vi "Test Clip.vi"() -> ()   [LabVIEW 2019, in "DAQmx.lvclass"]
uses:
  DAQmx.lvclass
  typedefs/DAQ.Config.AO.Range--enum.ctl
  <vilib>/measure/NI_MABase.lvlib
  <resource>/objmgr/daqmx.rc
panel:
  in  "AO.Range":T1
  in  "amplitude":dbl=1.0 format="%0.2p"
  in  "Numeric":i32=1
  out "x-y":dbl
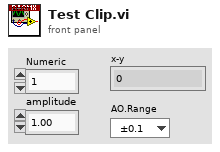
[diagram p1: front panel]
types:
  T1 = typedef "DAQmx.lvclass/DAQ.Config.AO.Range--enum.ctl" = enum16{"±0.1", "±1.0", "±3.5", "±10.0", ""}
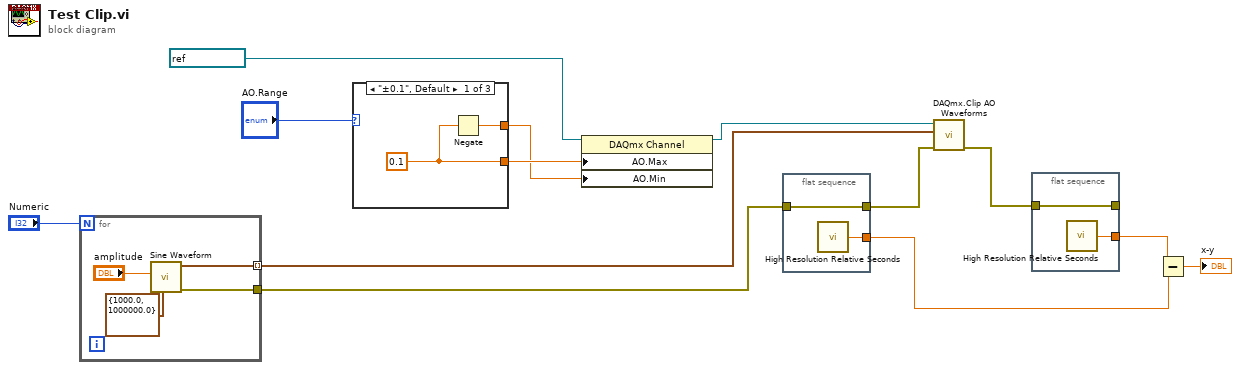
[diagram p0: block diagram]
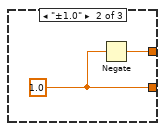
[diagram p2: hidden frame]
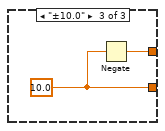
[diagram p3: hidden frame]
diagram:
  n1 = for {
    N: "Numeric" -> [_]
    tunnel: [w16] -> w11
    tunnel: [w15] -> w10 mode=indexing
    n2 = call <vilib>:"Sine Waveform.vi"("sampling info"=cluster{"Fs":dbl, "#s":dbl} {"Fs"=1000.0, "#s"=1000000.0}, "amplitude"="amplitude") -> ("error out"=w16:errorcluster, "signal out"=w15:waveform(dbl))  [unwired: 8 in]
  }
  n3 = case shown="\"±0.1\", Default" "AO.Range" {
    tunnel: [w19 w21 w23] -> w3
    tunnel: [w18 w20 w22] -> w2
    frame "±0.1", Default {
      w19 = 0.1
      n4 = Negate(x=w19) -> (-x=w18:dbl)
    }
    frame "±1.0" {
      w21 = 1.0
      n5 = Negate(x=w21) -> (-x=w20:dbl)
    }
    frame "±10.0" {
      w23 = 10.0
      n6 = Negate(x=w23) -> (-x=w22:dbl)
    }
  }
  n7 = property class="DAQmx Channel"(reference=refnum<k21> refnum ("task"), "AO.Max"=w3, "AO.Min"=w2) -> (reference out=w1:refnum<k21>)  [unwired: 1 in, 1 out]
  n8 = flat-sequence {
    tunnel: [w25] -> w12
    tunnel: w11 -> [w25]
    tunnel: [w24] -> w7
    frame #0 {
      n9 = call <vilib>:"High Resolution Relative Seconds.vi"() -> ("relative seconds"=w24:dbl)
    }
  }
  n10 = call "DAQmx.Clip AO Waveforms.vi"("error in (no error)"=w12, "AO []"=w10, "task"=w1) -> ("error out"=w9:errorcluster)  [unwired: 6 in, 2 out]
  n11 = flat-sequence {
    tunnel: [w27] -> _
    tunnel: w9 -> [w27]
    tunnel: [w26] -> w8
    frame #0 {
      n12 = call <vilib>:"High Resolution Relative Seconds.vi"() -> ("relative seconds"=w26:dbl)
    }
  }
  n13 = Subtract(x=w8, y=w7) -> (x-y=→"x-y":dbl)
